vi "Init.vi"(0 "Arduino Resource":T3={"VISA resource"="", "Board Type"=enum."Uno", "Connection Type"=enum."USB / Serial", "Bytes Per Packet (15)"=15}, 1 "Accel Full Scale Range":T2, 2 "Gyro Full Scale Range":T1, 5 "Device Address":T5=104 items=["0x68"=104, "0x69"=105], 9 "Clock Source":u8=1, 11 "error in (no error)":errorcluster) -> (4 "Arduino Resource":T3={"VISA resource"="", "Board Type"=enum."Uno", "Connection Type"=enum."USB / Serial", "Bytes Per Packet (15)"=15}, 15 "error out":errorcluster)   [LabVIEW 2012, in "LIFA MPU-60X0.lvlib"]
uses:
  LIFA MPU-60X0.lvlib
  <vilib>/LabVIEW Interface for Arduino/Type Defs/Arduino Resource.ctl
  <vilib>/LabVIEW Interface for Arduino/Type Defs/Board Type.ctl
  DeviceAddresses.ctl
  AccelFullScaleRanges.ctl
  GyroFullScaleRanges.ctl
  <vilib>/LabVIEW Interface for Arduino/LabVIEW Interface for Arduino.lvlib
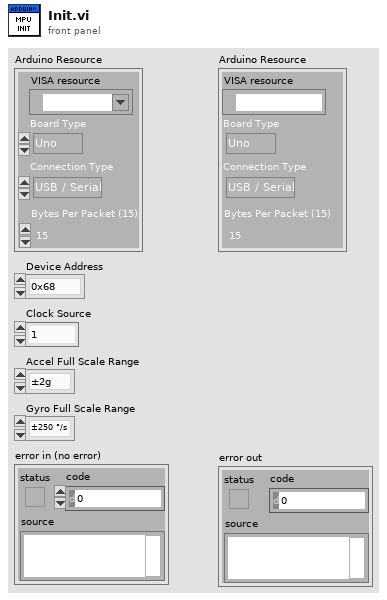
[diagram p1: front panel]
types:
  T1 = typedef "LIFA MPU-60X0.lvlib/GyroFullScaleRanges.ctl" = enum8{"±250 °/s", "±500 °/s", "±1000 °/s", "±2000 °/s"}
  T2 = typedef "LIFA MPU-60X0.lvlib/AccelFullScaleRanges.ctl" = enum16{"±2g", "±4g", "±8g", "±16g"}
  T3 = typedef "LabVIEW Interface for Arduino.lvlib/Arduino Resource.ctl" = cluster{"VISA resource":refnum<visa-resource-name>, "Board Type":T4, "Connection Type":enum8{"USB / Serial"}, "Bytes Per Packet (15)":u8}
  T4 = typedef "LabVIEW Interface for Arduino.lvlib/Board Type.ctl" = enum16{"Uno", "Dimuelanove w/Atmega 328", "Mega 2560"}
  T5 = typedef "LIFA MPU-60X0.lvlib/DeviceAddresses.ctl" = u8
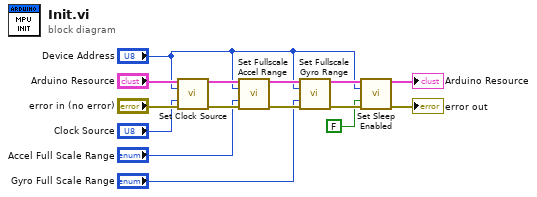
[diagram p0: block diagram]
diagram:
  n1 = call "Set Clock Source.vi"("Arduino Resource"="Arduino Resource", "Device Address"="Device Address", "Clock Source"="Clock Source", "error in (no error)"="error in (no error)") -> ("Arduino Resource"=w15:T3, "error out"=w9:errorcluster)  [unwired: 10 in]
  n2 = call "Set Fullscale Accel Range.vi"("Arduino Resource"=w15, "Device Address"="Device Address", "Accel Full Scale Range"="Accel Full Scale Range", "error in (no error)"=w9) -> ("Arduino Resource"=w14:T3, "error out"=w8:errorcluster)  [unwired: 10 in]
  n3 = call "Set Fullscale Gyro Range.vi"("Arduino Resource"=w14, "Device Address"="Device Address", "Gyro Full Scale Range"="Gyro Full Scale Range", "error in (no error)"=w8) -> ("Arduino Resource"=w13:T3, "error out"=w7:errorcluster)  [unwired: 10 in]
  n4 = call "Set Sleep Enabled.vi"("Arduino Resource"=w13, "Device Address"="Device Address", "Sleep?"=FALSE, "error in (no error)"=w7) -> ("Arduino Resource"=→"Arduino Resource":T3, "error out"=→"error out":errorcluster)  [unwired: 10 in]
